vi "Add Menu Item.vi"(8 "error in (no error)":errorcluster, 9 "Item":string, 11 "module in":refnum<class "Header.lvclass">) -> (0 "error out":errorcluster, 3 "module out":refnum<class "Header.lvclass">)   [LabVIEW 2024, in "Header.lvclass"]
uses:
  Header.lvclass
  Header.lvclass/Header.ctl
  C:/Git/JA/JQMH/RQMHCore/ModuleCore/Module.lvclass
  C:/Git/JA/JQMH/ModuleTemplates/Header/Header.lvclass
  RQMHCore/ModuleCore/Module.lvclass
  RQMHCore/ModuleCore/Reply.ctl
  Add Menu Item Args.ctl
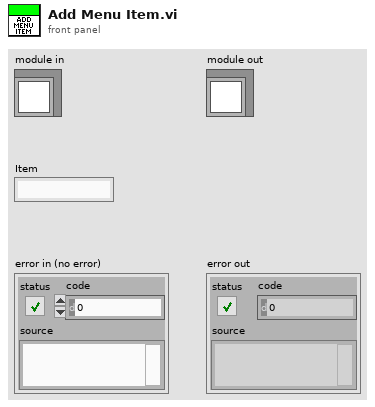
[diagram p1: front panel]
types:
  T1 = typedef "Header.lvclass/Add Menu Item Args.ctl" = cluster{"Item":string}
  T2 = typedef "Module.lvclass/Reply.ctl" = cluster{"Expects Reply":bool, "Reply":refnum<notifier>}
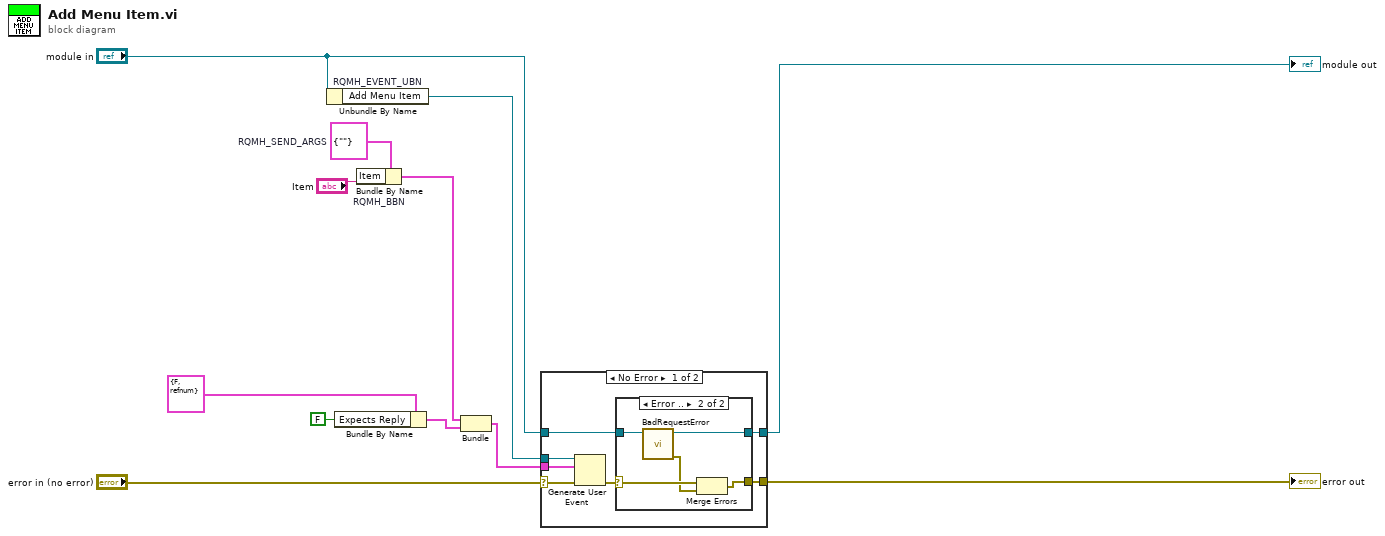
[diagram p0: block diagram]
diagram:
  w7 = T1 {"Item"=""}  # RQMH_SEND_ARGS
  n1 = Unbundle By Name "RQMH_EVENT_UBN"("module in") -> ("Add Menu Item"=w5:refnum<user-event>)
  n2 = Bundle By Name(cluster=T2 {"Expects Reply"=FALSE, "Reply"=refnum} ("Reply"), "Expects Reply"=FALSE) -> (w12:T2)
  n3 = Bundle By Name "RQMH_BBN"(cluster=w7, "Item"="Item") -> (w4:T1)
  n4 = Bundle("RQMH_SEND_ARGS"=w4, "Reply"=w12) -> (w11:cluster{"RQMH_SEND_ARGS":T1, "Reply":T2})  [unwired: 1 in]
  n5 = case shown="No Error" "error in (no error)" {
    selector: "error in (no error)" -> [w16 w27]
    tunnel: w11 -> [w19 _]
    tunnel: w5 -> [w18 _]
    tunnel: [w15 w27] -> w2
    tunnel: "module in" -> [w14 w28]
    tunnel: [w13 w28] -> w8
    frame No Error {
      n6 = Generate User Event(user event=w18, event data cluster=w19, error in=w16) -> (error out=w17:errorcluster)  [unwired: 1 in, 1 out]
      n7 = case shown="Error .." w17 {
        selector: w17 -> [w20 w26]
        tunnel: [w20 w25] -> w15
        tunnel: w14 -> [w21 w24]
        tunnel: [w21 w23] -> w13
        frame No Error {
        }
        frame Error {
          n8 = call "BadRequestError.vi"("JQMHModule in"=w24) -> ("error out"=w22:errorcluster, "JQMHModule out"=w23:refnum<class "Header.lvclass">)  [unwired: 9 in]
          n9 = Merge Errors(w26, w22) -> (w25:errorcluster)
        }
      }
    }
    frame Error {
    }
  }
  "error out" <- w2
  "module out" <- w8
